vi "FlatToRichgrpc_reflection_v1alpha_ServerReflectionRequest.vi"(5 "OutputClusterType":T1, 11 "InputCluster":T2) -> (3 "OutputCluster":T1)   [LabVIEW 2025, in "reflection_server.lvlib"]
uses:
  reflection_server.lvlib
  grpc_reflection_v1alpha_ServerReflectionRequest_Flat.ctl
  grpc_reflection_v1alpha_ExtensionRequest_Flat.ctl
  grpc_reflection_v1alpha_ServerReflectionRequest.ctl
  grpc_reflection_v1alpha_ServerReflectionRequest_message_request/grpc_reflection_v1alpha_ServerReflectionRequest_message_request.lvclass
  grpc_reflection_v1alpha_ServerReflectionRequest_message_request/grpc_reflection_v1alpha_ServerReflectionRequest_message_request.lvclass/grpc_reflection_v1alpha_ServerReflectionRequest_message_request.ctl
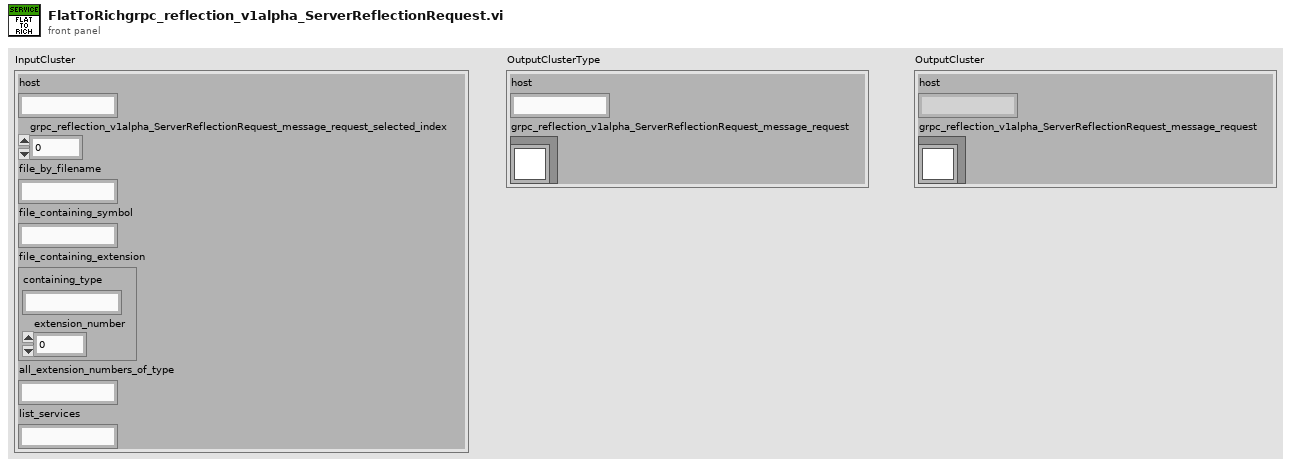
[diagram p1: front panel]
types:
  T1 = typedef "reflection_server.lvlib/grpc_reflection_v1alpha_ServerReflectionRequest.ctl" = cluster{"host":string, "grpc_reflection_v1alpha_ServerReflectionRequest_message_request":refnum<class "grpc_reflection_v1alpha_ServerReflectionRequest_message_request.lvclass">}
  T2 = typedef "reflection_server.lvlib/grpc_reflection_v1alpha_ServerReflectionRequest_Flat.ctl" = cluster{"host":string, "grpc_reflection_v1alpha_ServerReflectionRequest_message_request_selected_index":i32, "file_by_filename":string, "file_containing_symbol":string, "file_containing_extension":T3, "all_extension_numbers_of_type":string, "list_services":string}
  T3 = typedef "reflection_server.lvlib/grpc_reflection_v1alpha_ExtensionRequest_Flat.ctl" = cluster{"containing_type":string, "extension_number":i32}
  T4 = typedef "reflection_server.lvlib/grpc_reflection_v1alpha_ExtensionRequest.ctl" = cluster{"containing_type":string, "extension_number":i32}
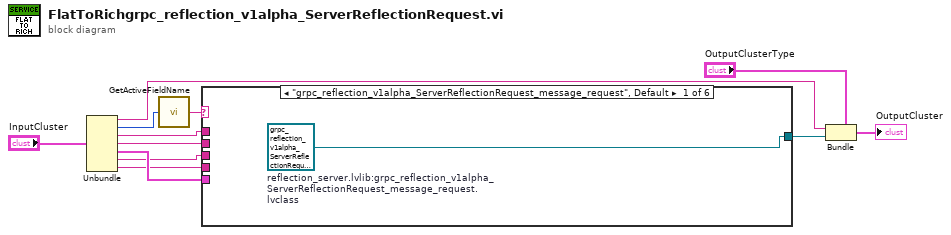
[diagram p0: block diagram]
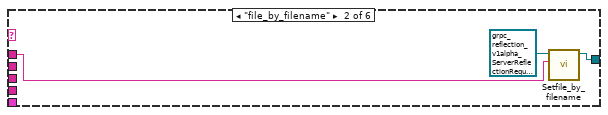
[diagram p2: hidden frame]
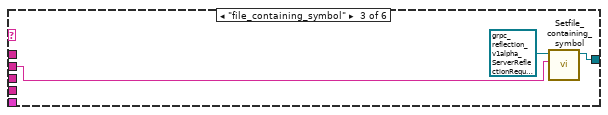
[diagram p3: hidden frame]
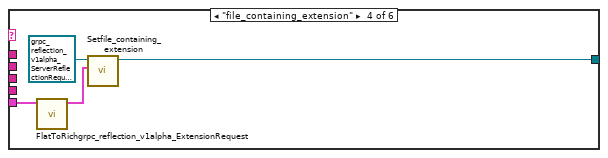
[diagram p4: hidden frame]
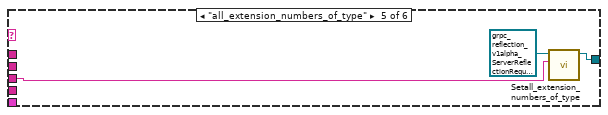
[diagram p5: hidden frame]
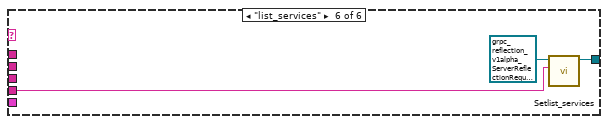
[diagram p6: hidden frame]
diagram:
  n1 = Unbundle "Unbundle"("InputCluster") -> ("host"=w9:string, "grpc_reflection_v1alpha_ServerReflectionRequest_message_request_selected_index"=w8:i32, "file_by_filename"=w5:string, "file_containing_symbol"=w4:string, "file_containing_extension"=w3:T3, "all_extension_numbers_of_type"=w2:string, "list_services"=w1:string)
  n2 = call "GetActiveFieldName.vi"("protobuf index"=w8) -> ("oneof field name"=w7:string)
  n3 = case "grpc_reflection_v1alpha_ServerReflectionRequest_message_request" shown="\"grpc_reflection_v1alpha_ServerReflectionRequest_message_request\", Default" w7 {
    tunnel: [w13 w15 w18 w21 w25 w28] -> w6
    tunnel: w5 -> [_ w16 _ _ _ _]
    tunnel: w4 -> [_ _ w19 _ _ _]
    tunnel: w3 -> [_ _ _ w23 _ _]
    tunnel: w2 -> [_ _ _ _ w26 _]
    tunnel: w1 -> [_ _ _ _ _ w29]
    frame "grpc_reflection_v1alpha_ServerReflectionRequest_message_request", Default {
      w13 = refnum<class "grpc_reflection_v1alpha_ServerReflectionRequest_message_request.lvclass"> refnum  # reflection_server.lvlib:grpc_reflection_v1alpha_ServerReflectionRequest_message_request.lvclass
    }
    frame "file_by_filename" {
      n4 = call "Setfile_by_filename.vi"("Set_Val"=w16, "OneOfTemplate in"=refnum<class "grpc_reflection_v1alpha_ServerReflectionRequest_message_request.lvclass"> refnum) -> ("OneOfTemplate out"=w15:refnum<class "grpc_reflection_v1alpha_ServerReflectionRequest_message_request.lvclass">)  [unwired: 8 in, 1 out]
    }
    frame "file_containing_symbol" {
      n5 = call "Setfile_containing_symbol.vi"("Set_Val"=w19, "OneOfTemplate in"=refnum<class "grpc_reflection_v1alpha_ServerReflectionRequest_message_request.lvclass"> refnum) -> ("OneOfTemplate out"=w18:refnum<class "grpc_reflection_v1alpha_ServerReflectionRequest_message_request.lvclass">)  [unwired: 8 in, 1 out]
    }
    frame "file_containing_extension" {
      n6 = call "FlatToRichgrpc_reflection_v1alpha_ExtensionRequest.vi"("InputCluster"=w23) -> ("OutputCluster"=w22:T4)  [unwired: 10 in]
      n7 = call "Setfile_containing_extension.vi"("Set_Val"=w22, "OneOfTemplate in"=refnum<class "grpc_reflection_v1alpha_ServerReflectionRequest_message_request.lvclass"> refnum) -> ("OneOfTemplate out"=w21:refnum<class "grpc_reflection_v1alpha_ServerReflectionRequest_message_request.lvclass">)  [unwired: 8 in, 1 out]
    }
    frame "all_extension_numbers_of_type" {
      n8 = call "Setall_extension_numbers_of_type.vi"("Set_Val"=w26, "OneOfTemplate in"=refnum<class "grpc_reflection_v1alpha_ServerReflectionRequest_message_request.lvclass"> refnum) -> ("OneOfTemplate out"=w25:refnum<class "grpc_reflection_v1alpha_ServerReflectionRequest_message_request.lvclass">)  [unwired: 8 in, 1 out]
    }
    frame "list_services" {
      n9 = call "Setlist_services.vi"("Set_Val"=w29, "OneOfTemplate in"=refnum<class "grpc_reflection_v1alpha_ServerReflectionRequest_message_request.lvclass"> refnum) -> ("OneOfTemplate out"=w28:refnum<class "grpc_reflection_v1alpha_ServerReflectionRequest_message_request.lvclass">)  [unwired: 8 in, 1 out]
    }
  }
  n10 = Bundle "Bundle"(cluster="OutputClusterType", "host"=w9, "grpc_reflection_v1alpha_ServerReflectionRequest_message_request"=w6) -> (→"OutputCluster":T1)
